vi "showOrHideByName.vi"(6 "showAll (F)":bool, 7 "visible? (T)":bool=TRUE, 9 "matchString":string, 11 "SceneObject in":refnum<vi>) -> (2 "matchedChildren":string[](array[string]))   [LabVIEW 2021]
panel:
  # "Iterates across the direct children of the supplied object and sets Alpha to 1 if matchString is found in child's name, else sets Alpha 0"
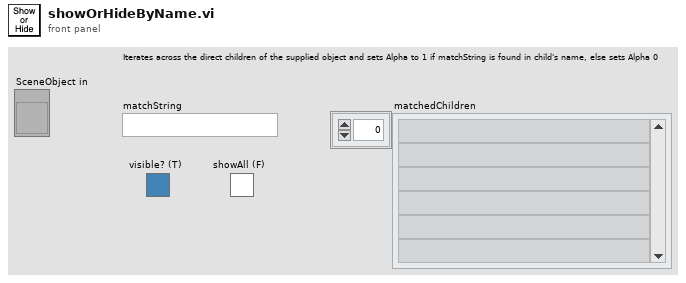
[diagram p1: front panel]
types:
  T1 = typedef "LVRGBAColorTypeDef.ctl" = cluster{"Red":sgl, "Green":sgl, "Blue":sgl, "Alpha":sgl}
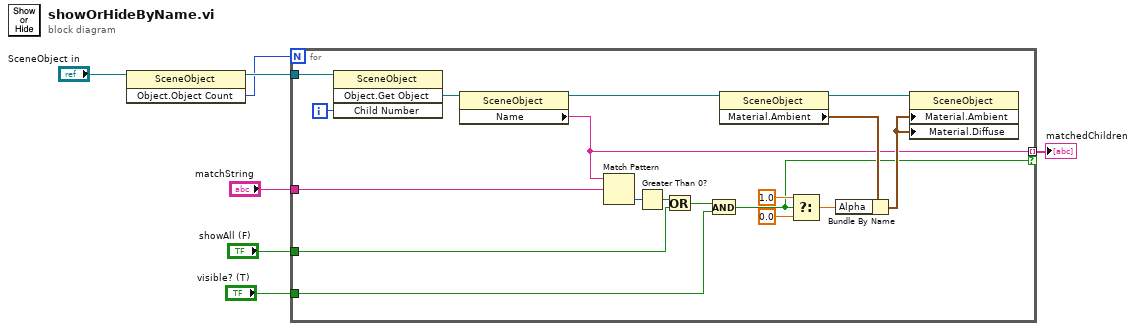
[diagram p0: block diagram]
diagram:
  n1 = invoke class="SceneObject" method="Object.Object Count"(reference="SceneObject in") -> (reference out=w5:refnum<vi>, "Child Count"=w4:i32)  [unwired: 2 in, 1 out]
  n2 = for {
    N: w4 -> [_]
    tunnel: w5 -> [w25]
    tunnel: "matchString" -> [w15]
    tunnel: "showAll (F)" -> [w12]
    tunnel: [w11] -> w2 mode=indexing if=w9
    tunnel: "visible? (T)" -> [w8]
    i -> [w24]
    n3 = invoke class="SceneObject" method="Object.Get Object"(reference=w25, "Child Number"=w24) -> ("Get Child"=w17:refnum<vi>)  [unwired: 2 in, 3 out]
    n4 = property class="SceneObject"(reference=w17) -> (reference out=w16:refnum<vi>, "Name"=w11:string)  [unwired: 1 in, 1 out]
    n5 = Match Pattern(string=w11, regular expression=w15) -> (offset past match=w14:i32)  [unwired: 1 in, 3 out]
    n6 = Greater Than 0?(x=w14) -> (x > 0?=w13:bool)
    n7 = Or(x=w13, y=w12) -> (x .or. y?=w10:bool)
    n8 = And(x=w10, y=w8) -> (x .and. y?=w9:bool)
    n9 = property class="SceneObject"(reference=w16) -> (reference out=w23:refnum<vi>, "Material.Ambient"=w22:T1)  [unwired: 1 in, 1 out]
    n10 = Select(t=1.0, s=w9, f=0.0) -> (s? t:f=w20:dbl)
    n11 = Bundle By Name(cluster=w22, "Alpha"=w20) -> (w21:T1)
    n12 = property class="SceneObject"(reference=w23, "Material.Ambient"=w21, "Material.Diffuse"=w21) -> ()  [unwired: 1 in, 2 out]
  }
  "matchedChildren" <- w2
